vi "test wire conversion.vi"() -> ()   [LabVIEW 2013, in "TEC tests.lvlib"]
uses:
  TEC tests.lvlib
  <vilib>/NI/Tag Bus Module Framework/channel/channel classification.ctl
  configuration/TEC configuration.lvclass
  <vilib>/NI/Tag Bus/table/data table.ctl
  <vilib>/NI/Tag Bus/dictionary/data dictionary.lvclass/data dictionary.ctl
  <vilib>/NI/Tag Bus Module Framework/channel/TBM channel.lvclass
  <vilib>/NI/Tag Bus Module Framework/root configuration/TBM configuration.lvclass
  <vilib>/NI/Tag Bus/dictionary/data dictionary.lvclass
  execution/TEC runtime.lvclass
  <vilib>/NI/Tag Bus/table/data table.lvlib
panel:
  out "x = y? fast":bool
  out "fast":errorcluster
  out "error out":errorcluster
  out "x = y?":bool
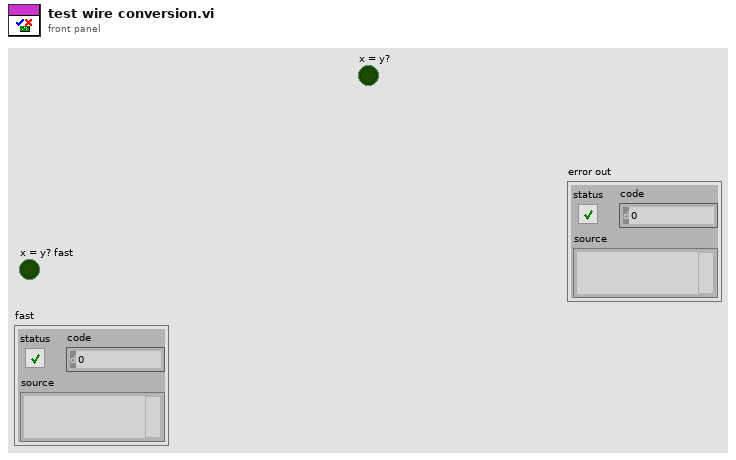
[diagram p1: front panel]
types:
  T1 = typedef "tag bus.lvlib/data table.lvlib/data table.ctl" = cluster{"Double":dbl[], "Single":sgl[], "I64":i64[], "I32":i32[], "I16":i16[], "I8":i8[], "U64":u64[], "U32":u32[], "U16":u16[], "U8":u8[], "Boolean":bool[], "String":string[], "Array of Double":cluster{"DBL Array":dbl[]}[], "Array of Single":cluster{"SGL Array":sgl[]}[], "Array of I64":cluster{"I64 Array":i64[]}[], "Array of I32":cluster{"I32 Array":i32[]}[], "Array of I16":cluster{"I16 Array":i16[]}[], "Array of I8":cluster{"I8 Array":i8[]}[], "Array of U64":cluster{"U64 Array":u64[]}[], "Array of U32":cluster{"U32 Array":u32[]}[], "Array of U16":cluster{"U16 Array":u16[]}[], "Array of U8":cluster{"U8 Array":u8[]}[], "Array of Boolean":cluster{"Boolean Array":bool[]}[], "Array of String":cluster{"String Array":string[]}[]}
  T2 = typedef "TBM channel.lvclass/channel classification.ctl" = enum16{"input data", "output data", "processing parameter", "processing result"}
  T3 = typedef "tag bus.lvlib/tag descriptor.lvclass/Data Type.ctl" = enum16{"Double", "Single", "I64", "I32", "I16", "I8", "U64", "U32", "U16", "U8", "Boolean", "String", "Array of Double", "Array of Single", "Array of I64", "Array of I32", "Array of I16", "Array of I8", "Array of U64", "Array of U32", "Array of U16", "Array of U8", "Array of Boolean", "Array of String"}
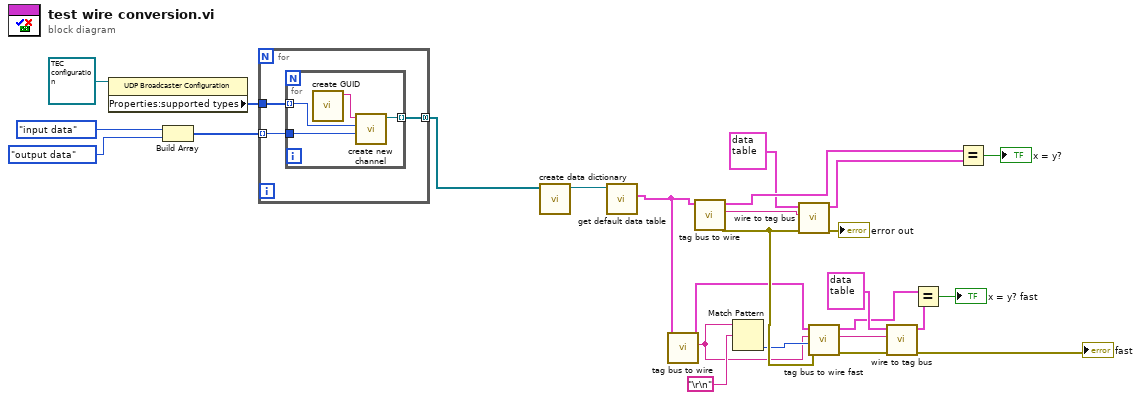
[diagram p0: block diagram]
diagram:
  n1 = property class="UDP Broadcaster Configuration"(reference=refnum<class "TEC configuration.lvclass"> refnum ("tag bus configurable plugin module configuration")) -> ("Properties:supported types"=w23:T3[])  [unwired: 1 in, 2 out]
  n2 = Build Array(channel_classification."input data" ("channel classification"), channel_classification."output data" ("channel classification")) -> (w24:T2[])
  n3 = for {
    tunnel: w24 -> [w29] mode=indexing
    tunnel: [w27] -> w20 mode=concatenating
    tunnel: w23 -> [w28]
    n4 = for {
      tunnel: w29 -> [w32]
      tunnel: [w33] -> w27 mode=indexing
      tunnel: w28 -> [w31] mode=indexing
      n5 = call <vilib>:"create GUID.vi"() -> ("uuid"=w30:string)  [unwired: 11 in]
      n6 = call <vilib>:"create new channel.vi"("channel classification"=w32, "data type"=w31, "channel name"=w30) -> ("channel"=w33:refnum<class "TBM channel.lvclass">)  [unwired: 8 in]
    }
  }
  n7 = call <vilib>:"create data dictionary.vi"("system tags"=w20) -> ("data dictionary"=w21:refnum<class "data dictionary.lvclass">)  [unwired: 9 in, 1 out]
  n8 = call <vilib>:"get default data table.vi"("data dictionary in"=w21) -> ("default data table"=w14:T1)  [unwired: 9 in, 1 out]
  n9 = call "tag bus to wire.vi"("data table in"=w14) -> ("wire data"=w1:string, "data table out"=w11:T1)  [unwired: 8 in, 1 out]
  n10 = call "tag bus to wire.vi"("data table in"=w14) -> ("error out"=w12:errorcluster, "wire data"=w19:string, "data table out"=w17:T1)  [unwired: 8 in]
  n11 = Match Pattern(string=w1, regular expression="\r\n") -> (offset past match=w3:i32)  [unwired: 1 in, 3 out]
  n12 = call "wire to tag bus.vi"("error in"=w12, "wire data"=w19, "data table in"=T1 {"Double"=[], "Single"=[], "I64"=[], "I32"=[], "I16"=[], "I8"=[], "U64"=[], "U32"=[], "U16"=[], "U8"=[], "Boolean"=[], "String"=[], "Array of Double"=[], "Array of Single"=[], "Array of I64"=[], "Array of I32"=[], "Array of I16"=[], "Array of I8"=[], "Array of U64"=[], "Array of U32"=[], "Array of U16"=[], "Array of U8"=[], "Array of Boolean"=[], "Array of String"=[]}) -> ("error out"=→"error out":errorcluster, "data table out"=w18:T1)  [unwired: 7 in]
  n13 = call "tag bus to wire fast.vi"("error in"=w12, "data index"=w3, "string allocation"=w1, "data table in"=w11) -> ("error out"=w9:errorcluster, "wire data"=w10:string, "data table out"=w5:T1)  [unwired: 5 in]
  n14 = call "wire to tag bus.vi"("error in"=w9, "wire data"=w10, "data table in"=T1 {"Double"=[5.0, 0.0, 0.0, 0.0, 0.0, 0.0, 0.0, 0.0, 0.0, 0.0, 0.0, 0.0, 0.0, 0.0, 0.0, 0.0, 0.0, 0.0, 0.0, 0.0, 0.0, 0.0, 0.0, 0.0, 0.0, 0.0, 0.0, 0.0, 0.0, 0.0, 0.0, 0.0, 0.0, 0.0, 0.0, 0.0, 0.0, 0.0, 0.0, 0.0, 0.0, 0.0, 0.0, 0.0, 0.0, 0.0, 0.0, 0.0, 0.0, 0.0, 0.0, 0.0, 0.0, 0.0, 0.0, 0.0, 0.0, 0.0, 0.0, 0.0, 0.0, 0.0, 0.0, 0.0, 0.0, 0.0, 0.0, 0.0, 0.0, 0.0, 0.0, 0.0, 0.0, 0.0, 0.0, 0.0, 0.0, 0.0, 0.0, 0.0, 0.0, 0.0, 0.0, 0.0, 0.0, 0.0, 0.0, 0.0, 0.0, 0.0, 0.0, 0.0, 0.0, 0.0, 0.0, 0.0, 0.0, 0.0, 0.0, 0.0], "Single"=[], "I64"=[], "I32"=[], "I16"=[], "I8"=[], "U64"=[], "U32"=[], "U16"=[], "U8"=[], "Boolean"=[], "String"=[], "Array of Double"=[], "Array of Single"=[], "Array of I64"=[], "Array of I32"=[], "Array of I16"=[], "Array of I8"=[], "Array of U64"=[], "Array of U32"=[], "Array of U16"=[], "Array of U8"=[], "Array of Boolean"=[], "Array of String"=[]}) -> ("error out"=→"fast":errorcluster, "data table out"=w4:T1)  [unwired: 7 in]
  n15 = Equal?(x=w5, y=w4) -> (x = y?=→"x = y? fast":bool)
  n16 = Equal?(x=w17, y=w18) -> (x = y?=→"x = y?":bool)
